vi "Dashboard Main.vi"() -> ()   [LabVIEW 2016]
uses:
  src/ConfigXML/typedefs/ConfigXMLInputData.ctl
  src/General/RemoteFiles/connectionData.ctl
  src/LoggerViewer/src/LoggerViewerInputData.ctl
  src/General/CorePluginInfo.ctl
panel:
  in  "stopButton":bool
  in  "MainDashTab":T1(tab)
  in  "VisionConfig":T2={"BasePath"=path "C:/CustomDashboard/VisionConfig", "CommunicationData"={"TargetFilePath"="/media/sda1", "ConnectionData"={"host"="roborio-223-frc.local", "user"="lvuser", "password"="", "port"=22}}}
  in  "Robo Logger":T4={"ConnectionData"={"host"="roborio-223-frc.local", "user"="lvuser", "password"="", "port"=5808}, "BasePath"=path "C:/CustomDashboard/RoboLogger", "remotePath"="/media/sda1/logging", "Console buffer size"=25000, "remoteLoggerPort"=5801}
  in  "Main Config":T2={"BasePath"=path "C:/CustomDashboard/MainConfig", "CommunicationData"={"TargetFilePath"="/media/sda1", "ConnectionData"={"host"="roborio-223-frc.local", "user"="lvuser", "password"="", "port"=22}}}
  out "Robot IP":string
  in  "Window Docked":bool
  in  "VisionViewer":T3
  in  "AutoConfig":T2={"BasePath"=path "C:/CustomDashboard/VisionConfig", "CommunicationData"={"TargetFilePath"="/media/sda1", "ConnectionData"={"host"="roborio-223-frc.local", "user"="lvuser", "password"="", "port"=22}}}
  out "TeleopImageDisplay":T5(plugin-control)
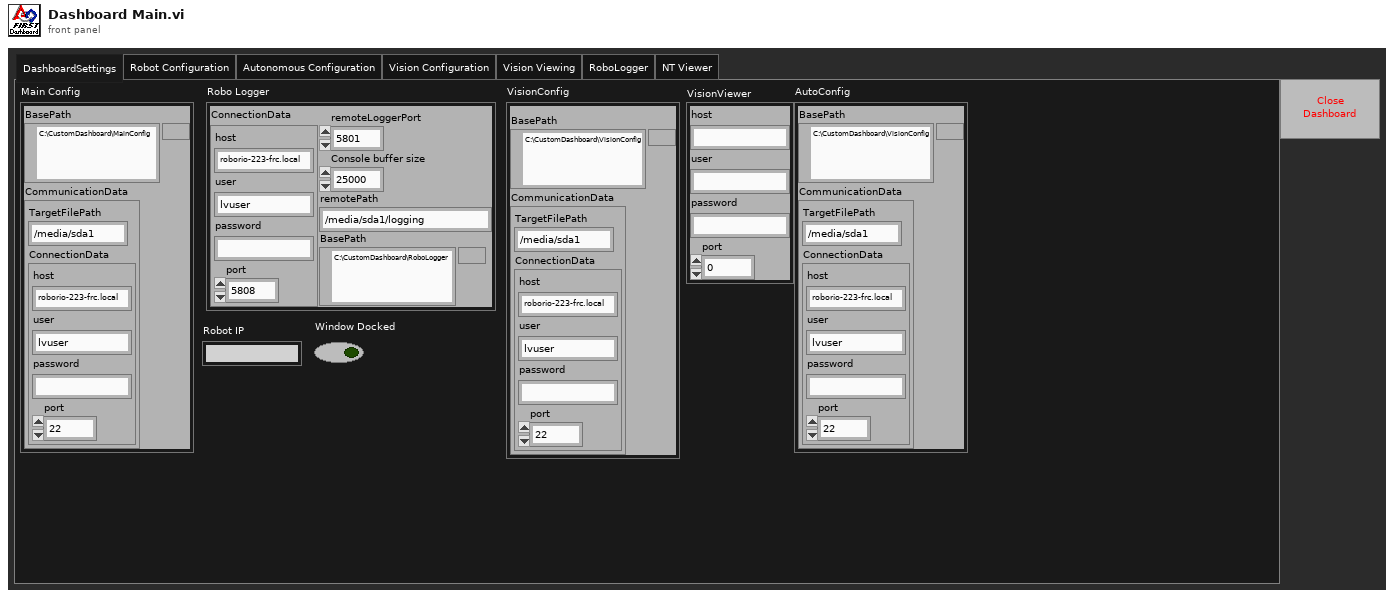
[diagram p1: front panel]
types:
  T1 = enum32{"DashboardSettings", "Robot Configuration", "Autonomous Configuration", "Vision Configuration", "Vision Viewing", "Teleop", "RoboLogger", "NT Viewer"}
  T2 = typedef "ConfigXMLInputData.ctl" = cluster{"BasePath":path, "CommunicationData":cluster{"TargetFilePath":string, "ConnectionData":T3}}
  T3 = typedef "connectionData.ctl" = cluster{"host":string, "user":string, "password":string, "port":u16}
  T4 = typedef "LoggerViewerInputData.ctl" = cluster{"ConnectionData":T3, "BasePath":path, "remotePath":string, "Console buffer size":u32, "remoteLoggerPort":u16}
  T5 = typedef "IMAQ Image.ctl" = refnum<image>
  T6 = typedef "CorePluginInfo.ctl" = cluster{"Notifiers":cluster{"Robot IP Notifier":refnum<notifier>, "Window Mode Notifier":refnum<notifier>, "Stop Notifier":refnum<notifier>}}
  T7 = cluster{refnum<vi>, "NT Viewer Panel":refnum<vi>}
  T8 = cluster{refnum<vi>, "NT Viewer Panel":refnum<vi>}[]
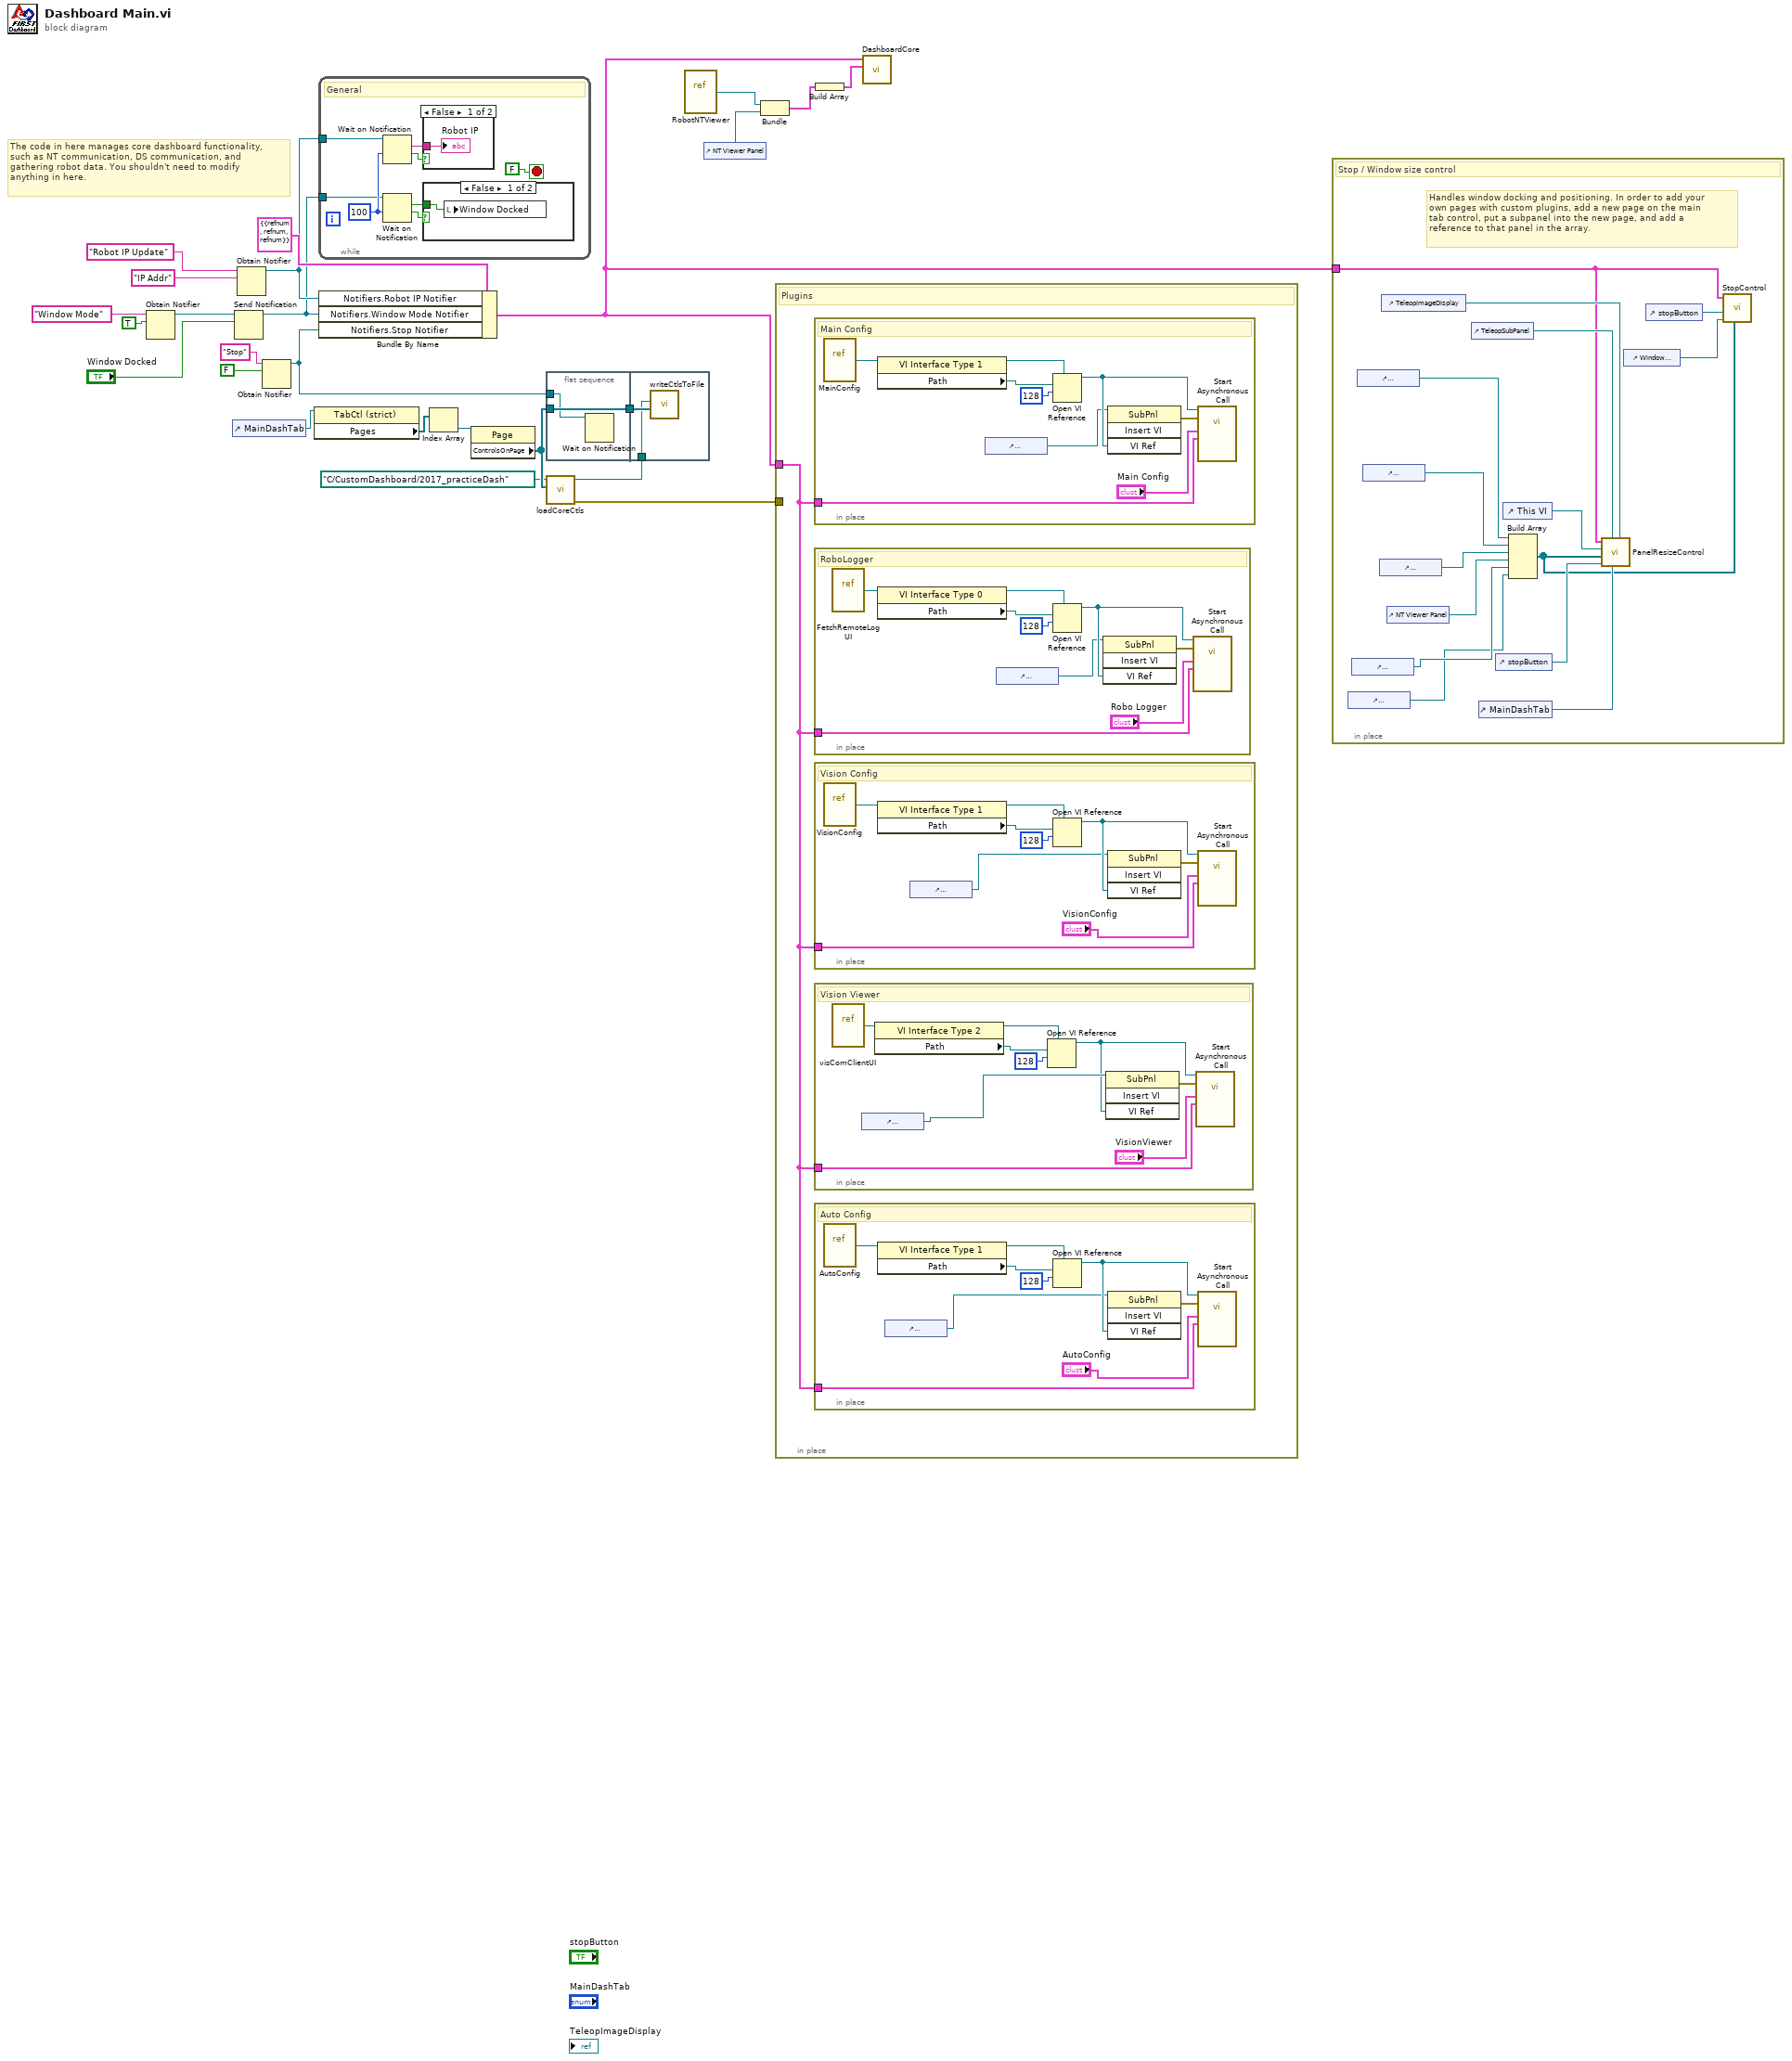
[diagram p0: block diagram]
diagram:
  # "The code in here manages core dashboard functionality, \nsuch as NT communication, DS communication, and \ngathering robot data. You shouldn't need to modify \nanything in here."
  n1 = Obtain Notifier(name (unnamed)="Window Mode", notification data type=TRUE) -> (notifier out=w15:refnum<notifier>)  [unwired: 2 in, 2 out]
  n2 = control-ref of="MainDashTab"() -> (w23:refnum<vi>)
  n3 = Send Notification(notification="Window Docked", notifier=w15) -> (notifier out=w12:refnum<notifier>)  [unwired: 1 in, 1 out]
  n4 = Obtain Notifier(name (unnamed)="Robot IP Update", notification data type="IP Addr" ("name (unnamed)")) -> (notifier out=w13:refnum<notifier>)  [unwired: 2 in, 2 out]
  n5 = Obtain Notifier(name (unnamed)="Stop", notification data type=FALSE) -> (notifier out=w8:refnum<notifier>)  [unwired: 2 in, 2 out]
  n6 = property class="TabCtl (strict)"(reference=w23) -> ("Pages"=w24:refnum<vi>[])  [unwired: 1 in, 2 out]
  n7 = while {
    tunnel: w13 -> [w32]
    tunnel: w12 -> [w26]
    stop <- FALSE stop-if-true
    w29 = 100 ("timeout in ms (-1)")
    # "General"
    n8 = Wait on Notification(notifier=w32, timeout in ms (-1)=w29) -> (notification=w30:string, timed out?=w31:bool)  [unwired: 2 in, 2 out]
    n9 = Wait on Notification(notifier=w26, timeout in ms (-1)=w29) -> (notification=w27:bool, timed out?=w28:bool)  [unwired: 2 in, 2 out]
    n10 = case shown="False" w31 {
      tunnel: w30 -> [w35 _]
      frame False {
        "Robot IP" <- w35
      }
      frame True {
      }
    }
    n11 = case shown="False" w28 {
      tunnel: w27 -> [w34 _]
      frame False {
        n12 = local write "Window Docked"(w34) -> ()
      }
      frame True {
      }
    }
  }
  n13 = Bundle By Name(cluster=T6 {"Notifiers"={"Robot IP Notifier"=refnum, "Window Mode Notifier"=refnum, "Stop Notifier"=refnum}} ("Plugin Info"), "Notifiers.Robot IP Notifier"=w13, "Notifiers.Window Mode Notifier"=w12, "Notifiers.Stop Notifier"=w8) -> (w25:T6)
  n14 = Index Array(array=w24) -> (element=w6:refnum<vi>)  [unwired: 1 in]
  n15 = property class="Page"(reference=w6) -> ("ControlsOnPage"=w10:refnum<vi>[])  [unwired: 1 in, 2 out]
  n16 = flat-sequence {
    tunnel: [w37] -> w11
    tunnel: w10 -> [w37]
    tunnel: w8 -> [w36]
    tunnel: w11 -> [w39]
    tunnel: w5 -> [w38]
    frame #0 {
      n17 = Wait on Notification(notifier=w36) -> ()  [unwired: 3 in, 4 out]
    }
    frame #1 {
      n18 = call "writeCtlsToFile.vi"("ControlsToSave"=w39, "path"=w38) -> ()  [unwired: 8 in, 2 out]
    }
  }
  n19 = call "loadCoreCtls.vi"("ControlsOnPage"=w10, "Base path"=path "C:/CustomDashboard/2017_practiceDash") -> ("error out"=w7:errorcluster, "path out"=w5:path)  [unwired: 8 in]
  n20 = vi-ref "RobotNTViewer.vi"() -> (w2:refnum<vi>)
  n21 = control-ref of="NT Viewer Panel"() -> (w1:refnum<vi>)
  n22 = Bundle(w2, "NT Viewer Panel"=w1) -> (w3:T7)  [unwired: 1 in]
  n23 = in-place {
    in-place-border: w25 -> [w40]
    in-place-border: w7 -> [_]
    # "Plugins"
    n24 = in-place {
      in-place-border: w40 -> [w70]
      # "Main Config"
      n25 = vi-ref "MainConfig.vi"() -> (w68:refnum<vi>)
      n26 = property class="VI Interface Type 1"(reference=w68) -> (reference out=w73:refnum<vi>, "Path"=w74:path)  [unwired: 1 in, 1 out]
      n27 = control-ref of="MainConfigSubPanel"() -> (w71:refnum<vi>)
      n28 = Open VI Reference(type specifier VI Refnum (for type only)=w73, vi path=w74, options=128) -> (vi reference=w76:refnum<vi>)  [unwired: 3 in, 1 out]
      n29 = invoke class="SubPnl" method="Insert VI"(reference=w71, "VI Ref"=w76) -> (error out=w75:errorcluster)  [unwired: 2 in, 3 out]
      n30 = call-by-ref "Start Asynchronous Call"(reference=w76, error in=w75, "Plugin info"=w70, "Input Data"="Main Config") -> ()  [unwired: 10 in, 2 out]
    }
    n31 = in-place {
      in-place-border: w40 -> [w77]
      # "RoboLogger"
      n32 = vi-ref "FetchRemoteLogUI.vi"() -> (w79:refnum<vi>)
      n33 = property class="VI Interface Type 0"(reference=w79) -> (reference out=w82:refnum<vi>, "Path"=w83:path)  [unwired: 1 in, 1 out]
      n34 = control-ref of="RoboLoggerPanel"() -> (w80:refnum<vi>)
      n35 = Open VI Reference(type specifier VI Refnum (for type only)=w82, vi path=w83, options=128) -> (vi reference=w85:refnum<vi>)  [unwired: 3 in, 1 out]
      n36 = invoke class="SubPnl" method="Insert VI"(reference=w80, "VI Ref"=w85) -> (error out=w84:errorcluster)  [unwired: 2 in, 3 out]
      n37 = call-by-ref "Start Asynchronous Call"(reference=w85, error in=w84, "Plugin Info"=w77, "Remote Logger Input Data"="Robo Logger") -> ()  [unwired: 10 in, 2 out]
    }
    n38 = in-place {
      in-place-border: w40 -> [w62]
      # "Vision Config"
      n39 = vi-ref "VisionConfig.vi"() -> (w61:refnum<vi>)
      n40 = property class="VI Interface Type 1"(reference=w61) -> (reference out=w64:refnum<vi>, "Path"=w65:path)  [unwired: 1 in, 1 out]
      n41 = control-ref of="VisionConfigSubPanel"() -> (w59:refnum<vi>)
      n42 = Open VI Reference(type specifier VI Refnum (for type only)=w64, vi path=w65, options=128) -> (vi reference=w67:refnum<vi>)  [unwired: 3 in, 1 out]
      n43 = invoke class="SubPnl" method="Insert VI"(reference=w59, "VI Ref"=w67) -> (error out=w66:errorcluster)  [unwired: 2 in, 3 out]
      n44 = call-by-ref "Start Asynchronous Call"(reference=w67, error in=w66, "Plugin info"=w62, "Input Data"="VisionConfig") -> ()  [unwired: 10 in, 2 out]
    }
    n45 = in-place {
      in-place-border: w40 -> [w53]
      # "Vision Viewer"
      n46 = vi-ref "visComClientUI.vi"() -> (w54:refnum<vi>)
      n47 = control-ref of="VisionViewerSubPanel"() -> (w51:refnum<vi>)
      n48 = property class="VI Interface Type 2"(reference=w54) -> (reference out=w56:refnum<vi>, "Path"=w57:path)  [unwired: 1 in, 1 out]
      n49 = Open VI Reference(type specifier VI Refnum (for type only)=w56, vi path=w57, options=128) -> (vi reference=w50:refnum<vi>)  [unwired: 3 in, 1 out]
      n50 = invoke class="SubPnl" method="Insert VI"(reference=w51, "VI Ref"=w50) -> (error out=w58:errorcluster)  [unwired: 2 in, 3 out]
      n51 = call-by-ref "Start Asynchronous Call"(reference=w50, error in=w58, "Plugin Info"=w53, "ConnectionData"="VisionViewer") -> ()  [unwired: 10 in, 2 out]
    }
    n52 = in-place {
      in-place-border: w40 -> [w44]
      # "Auto Config"
      n53 = vi-ref "AutoConfig.vi"() -> (w43:refnum<vi>)
      n54 = property class="VI Interface Type 1"(reference=w43) -> (reference out=w46:refnum<vi>, "Path"=w47:path)  [unwired: 1 in, 1 out]
      n55 = control-ref of="AutoConfigSubPanel"() -> (w41:refnum<vi>)
      n56 = Open VI Reference(type specifier VI Refnum (for type only)=w46, vi path=w47, options=128) -> (vi reference=w49:refnum<vi>)  [unwired: 3 in, 1 out]
      n57 = invoke class="SubPnl" method="Insert VI"(reference=w41, "VI Ref"=w49) -> (error out=w48:errorcluster)  [unwired: 2 in, 3 out]
      n58 = call-by-ref "Start Asynchronous Call"(reference=w49, error in=w48, "Plugin info"=w44, "Input Data"="AutoConfig") -> ()  [unwired: 10 in, 2 out]
    }
  }
  n59 = Build Array(w3) -> (w4:T8)
  n60 = call "DashboardCore.vi"("NT Viewer VIs"=w4, "Plugin Info"=w25) -> ()  [unwired: 10 in]
  n61 = in-place {
    in-place-border: w25 -> [w88]
    # "Handles window docking and positioning. In order to add your\nown pages with custom plugins, add a new page on the main\ntab control, put a subpanel into the new page, and add a\nreference to that panel in the array."
    # "Stop / Window size control"
    n62 = control-ref of="AutoConfigSubPanel"() -> (w86:refnum<vi>)
    n63 = control-ref of="VisionViewerSubPanel"() -> (w87:refnum<vi>)
    n64 = control-ref of="VisionConfigSubPanel"() -> (w100:refnum<vi>)
    n65 = control-ref of="MainConfigSubPanel"() -> (w99:refnum<vi>)
    n66 = control-ref of="RoboLoggerPanel"() -> (w93:refnum<vi>)
    n67 = control-ref of="TeleopImageDisplay"() -> (w94:refnum<vi>)
    n68 = control-ref of="NT Viewer Panel"() -> (w92:refnum<vi>)
    n69 = control-ref of="TeleopSubPanel"() -> (w95:refnum<vi>)
    n70 = control-ref of="MainDashTab"() -> (w97:refnum<vi>)
    n71 = control-ref of="stopButton"() -> (w98:refnum<vi>)
    n72 = control-ref of="This VI"() -> (w96:refnum<vi>)
    n73 = Build Array(w100, w99, w93, w92, w87, w86) -> (w89:refnum<vi>[])
    n74 = call "PanelResizeControl.vi"("TeleopDisplay"=w94, "MainDashTab"=w97, "TeleopSubPanel"=w95, "stopButton"=w98, "SubPanels"=w89, "TopLevelVI"=w96, "Plugin Info"=w88) -> ()  [unwired: 5 in]
    n75 = control-ref of="Window Docked"() -> (w90:refnum<vi>)
    n76 = control-ref of="stopButton"() -> (w91:refnum<vi>)
    n77 = call "StopControl.vi"("SubPanels"=w89, "WindowButton"=w90, "StopButton"=w91, "Plugin Info"=w88) -> ()  [unwired: 8 in]
  }
